vi "Periodic Tasks.vi"(8 "error in":errorcluster) -> ()   [LabVIEW 2013]
doc: "This VI runs in parallel to other tasks. It can contain as many user-defined periodic loops as you need. These can carry out PID or other sorts of timed response."
uses:
  <vilib>/Rock Robotics/SystemInterfaces/Utilities/FPGA_UtilitiesLED Source.ctl
  <vilib>/Rock Robotics/SystemInterfaces/Utilities/FPGA_UtilitiesLED State.ctl
  <vilib>/Rock Robotics/WPI/DriverStation/DriverStationLCD/WPI_DriverStationLCDLCDLine.ctl
  Robot Global Data.vi
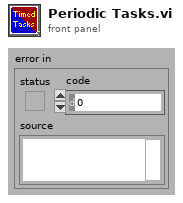
[diagram p1: front panel]
types:
  T1 = typedef "WPI_AnalogChannelDevRef.ctl" = cluster{"DevStatus":errorcluster, "Analog Module":T2, "Analog Channel":T3}
  T2 = typedef "FPGA_TypedefAnalogModule.ctl" = enum16{"Analog Module 1", "Analog Module 2"}
  T3 = typedef "FPGA_AIChannel.ctl" = enum8{"AI 1", "AI 2", "AI 3", "AI 4", "AI 5", "AI 6", "AI 7", "AI 8", "Invalid"}
  T4 = typedef "WPI_DigitalInputDevRef.ctl" = cluster{"DevStatus":errorcluster, "DIO Channel":T5, "Digital Module":T6}
  T5 = typedef "FPGA_DIOChannel.ctl" = enum8{"DIO 1", "DIO 2", "DIO 3", "DIO 4", "DIO 5", "DIO 6", "DIO 7", "DIO 8", "DIO 9", "DIO 10", "DIO 11", "DIO 12", "DIO 13", "DIO 14", "Invalid"}
  T6 = typedef "FPGA_TypedefDigitalModule.ctl" = enum16{"Digital Module 1", "Digital Module 2"}
  T7 = typedef "WPI_EncoderDevRef.ctl" = cluster{"DevStatus":errorcluster, "EncoderIndex":T8, "CounterIndex":T9, "DistancePerCount":dbl, "Decoding Type":T10}
  T8 = typedef "FPGA_EncoderIdx.ctl" = enum8{"Enc 0", "Enc 1", "Enc 2", "Enc 3", "Invalid"}
  T9 = typedef "FPGA_CounterCtrSystemIndex.ctl" = enum8{"Ctr 0", "Ctr 1", "Ctr 2", "Ctr 3", "Ctr 4", "Ctr 5", "Ctr 6", "Ctr 7", "Invalid"}
  T10 = typedef "WPI_EncoderType.ctl" = enum16{"1x", "2x", "4x"}
  T11 = cluster{"Winch Desired Location":dbl, "Winch Desired Location 2":dbl, "Winch Desired Location 3":dbl}
  T12 = typedef "FPGA_UtilitiesLED State.ctl" = enum16{"Off", "On", "Toggle"}
  T13 = typedef "FPGA_UtilitiesLED Source.ctl" = enum16{"User LED", "FPGA LED"}
  T14 = typedef "WPI_DriverStationLCDLCDLine.ctl" = enum16{"Main - Line 1", "User - Line 2", "User - Line 3", "User - Line 4", "User - Line 5", "User - Line 6"}
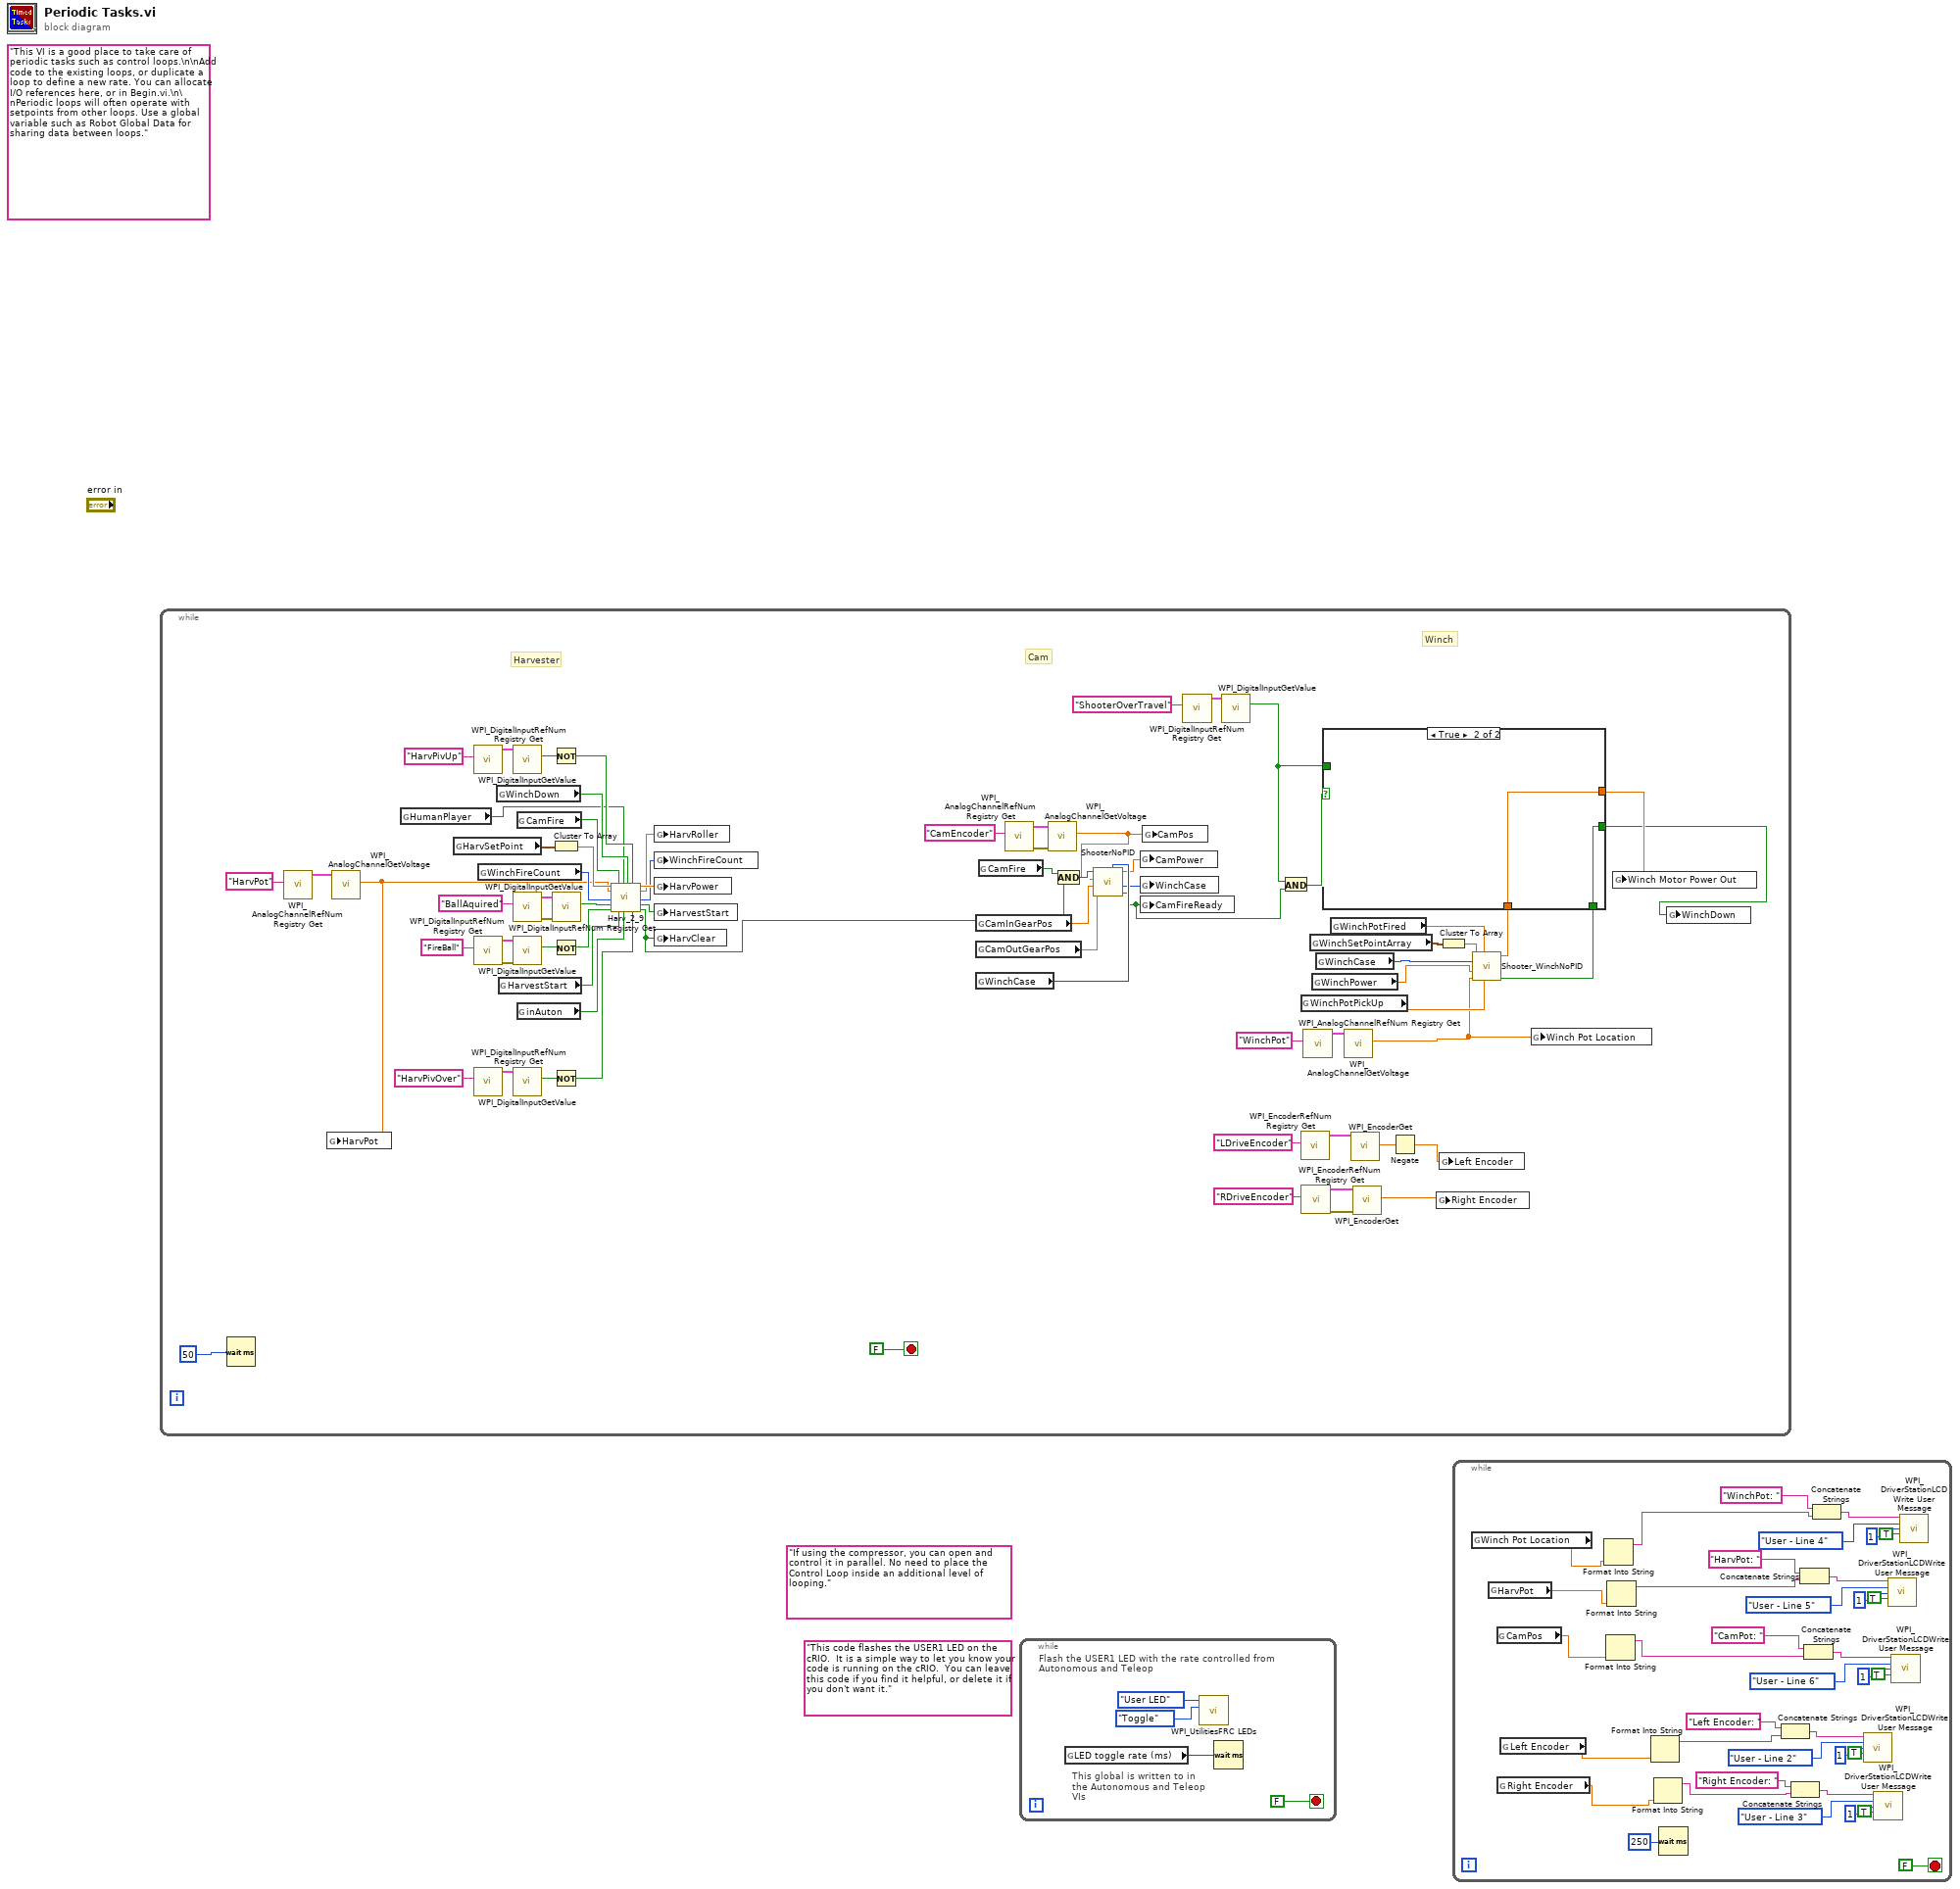
[diagram p0: block diagram]
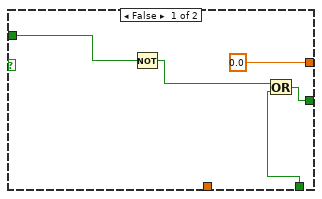
[diagram p2: hidden frame]
diagram:
  (unwired) "If using the compressor, you can open and control it in parallel. No need to place the Control Loop inside an additional level of looping."
  (unwired) "This code flashes the USER1 LED on the cRIO.  It is a simple way to let you know your code is running on the cRIO.  You can leave this code if you find it helpful, or delete it if you don't want it."
  (unwired) "This VI is a good place to take care of periodic tasks such as control loops.\n\nAdd code to the existing loops, or duplicate a loop to define a new rate. You can allocate I/O references here, or in Begin.vi.\n\nPeriodic loops will often operate with setpoints from other loops. Use a global variable such as Robot Global Data for sharing data between loops."
  n1 = while {
    stop <- FALSE stop-if-true
    # "Winch"
    # "Cam"
    # "Harvester"
    n2 = Wait (ms)(milliseconds to wait=u32 50) -> ()  [unwired: 1 out]
    n3 = call <vilib>:"WPI_AnalogChannelRefNum Registry Get.vi"("refnum name"="HarvPot") -> ("AIDeviceRef"=w71:T1)  [unwired: 9 in, 1 out]
    n4 = call <vilib>:"WPI_AnalogChannelGetVoltage.vi"("AIDeviceRef"=w71) -> ("Voltage"=w10:dbl)  [unwired: 8 in, 2 out]
    n5 = global write "Robot Global Data.vi" "HarvPot"(w10) -> ()
    n6 = global read "Robot Global Data.vi" "HumanPlayer"() -> (w1:bool)
    n7 = global read "Robot Global Data.vi" "HarvSetPoint"() -> (w38:cluster{"Out":dbl, "In":dbl, "Clear":dbl})
    n8 = call <vilib>:"WPI_DigitalInputRefNum Registry Get.vi"("refnum name"="HarvPivUp") -> ("DigitalInputDevRef"=w55:T4)  [unwired: 9 in, 1 out]
    n9 = call <vilib>:"WPI_DigitalInputRefNum Registry Get.vi"("refnum name"="FireBall") -> ("error out"=w44:errorcluster, "DigitalInputDevRef"=w45:T4)  [unwired: 9 in]
    n10 = call <vilib>:"WPI_DigitalInputRefNum Registry Get.vi"("refnum name"="HarvPivOver") -> ("DigitalInputDevRef"=w63:T4)  [unwired: 9 in, 1 out]
    n11 = global read "Robot Global Data.vi" "WinchFireCount"() -> (w13:i32)
    n12 = global read "Robot Global Data.vi" "WinchDown"() -> (w31:bool)
    n13 = global read "Robot Global Data.vi" "HarvestStart"() -> (w42:bool)
    n14 = call <vilib>:"WPI_DigitalInputGetValue.vi"("DigitalInputDevRef"=w55) -> ("Value"=w34:bool)  [unwired: 8 in, 2 out]
    n15 = call <vilib>:"WPI_DigitalInputRefNum Registry Get.vi"("refnum name"="BallAquired") -> ("error out"=w51:errorcluster, "DigitalInputDevRef"=w50:T4)  [unwired: 9 in]
    n16 = call <vilib>:"WPI_DigitalInputGetValue.vi"("error in (no error)"=w44, "DigitalInputDevRef"=w45) -> ("Value"=w41:bool)  [unwired: 7 in, 2 out]
    n17 = call <vilib>:"WPI_DigitalInputGetValue.vi"("DigitalInputDevRef"=w63) -> ("Value"=w36:bool)  [unwired: 8 in, 2 out]
    n18 = global read "Robot Global Data.vi" "CamFire"() -> (w43:bool)
    n19 = global read "Robot Global Data.vi" "inAuton"() -> (w15:bool)
    n20 = Not(x=w34) -> (.not. x?=w33:bool)
    n21 = Cluster To Array(cluster=w38) -> (array=w37:dbl[])
    n22 = call <vilib>:"WPI_DigitalInputGetValue.vi"("error in (no error)"=w51, "DigitalInputDevRef"=w50) -> ("Value"=w40:bool)  [unwired: 7 in, 2 out]
    n23 = Not(x=w41) -> (.not. x?=w39:bool)
    n24 = Not(x=w36) -> (.not. x?=w35:bool)
    n25 = call "Harv_2_9.vi"("HarvSetpoints"=w37, "HarvPot"=w10, "Count"=w13, "BallAcquired"=w40, "FireBallSen"=w39, "Fire"=w43, "Harvest"=w42, "HPButton"=w1, "inAuton?"=w15, "WinchDown"=w31, "HarvPivUP"=w33, "HarvPivPickupLim"=w35) -> ("HarvPower"=w48:dbl, "HarvRoller"=w47:dbl, "CountOut"=w12:i32, "HarvStart"=w32:bool, "HarvCleared"=w5:bool)  [unwired: 3 in]
    n26 = global write "Robot Global Data.vi" "HarvRoller"(w47) -> ()
    n27 = global write "Robot Global Data.vi" "WinchFireCount"(w12) -> ()
    n28 = global write "Robot Global Data.vi" "HarvPower"(w48) -> ()
    n29 = global write "Robot Global Data.vi" "HarvestStart"(w32) -> ()
    n30 = global write "Robot Global Data.vi" "HarvClear"(w5) -> ()
    n31 = global read "Robot Global Data.vi" "CamInGearPos"() -> (w20:dbl)
    n32 = global read "Robot Global Data.vi" "CamOutGearPos"() -> (w19:dbl)
    n33 = global read "Robot Global Data.vi" "WinchCase"() -> (w21:i32)
    n34 = global read "Robot Global Data.vi" "CamFire"() -> (w57:bool)
    n35 = call <vilib>:"WPI_AnalogChannelRefNum Registry Get.vi"("refnum name"="CamEncoder") -> ("error out"=w59:errorcluster, "AIDeviceRef"=w58:T1)  [unwired: 9 in]
    n36 = call <vilib>:"WPI_AnalogChannelGetVoltage.vi"("error in (no error)"=w59, "AIDeviceRef"=w58) -> ("Voltage"=w9:dbl)  [unwired: 7 in, 2 out]
    n37 = And(x=w57, y=w5) -> (x .and. y?=w22:bool)
    n38 = call "ShooterNoPID.vi"("WinchCaseIn"=w21, "InGearPosLow"=w19, "InGearPosHigh"=w20, "Pot"=w9, "Fire"=w22) -> ("There?"=w16:bool, "WinchCase"=w17:i32, "Power"=w18:dbl)  [unwired: 4 in]
    n39 = global write "Robot Global Data.vi" "CamPower"(w18) -> ()
    n40 = global write "Robot Global Data.vi" "WinchCase"(w17) -> ()
    n41 = global write "Robot Global Data.vi" "CamFireReady"(w16) -> ()
    n42 = global write "Robot Global Data.vi" "CamPos"(w9) -> ()
    n43 = call <vilib>:"WPI_DigitalInputRefNum Registry Get.vi"("refnum name"="ShooterOverTravel") -> ("DigitalInputDevRef"=w54:T4)  [unwired: 9 in, 1 out]
    n44 = call <vilib>:"WPI_DigitalInputGetValue.vi"("DigitalInputDevRef"=w54) -> ("Value"=w30:bool)  [unwired: 8 in, 2 out]
    n45 = And(x=w30, y=w16) -> (x .and. y?=w52:bool)
    n46 = global read "Robot Global Data.vi" "WinchPotPickUp"() -> (w14:dbl)
    n47 = call <vilib>:"WPI_EncoderRefNum Registry Get.vi"("refnum name"="LDriveEncoder") -> ("EncoderDevRef"=w65:T7)  [unwired: 9 in, 1 out]
    n48 = call <vilib>:"WPI_EncoderRefNum Registry Get.vi"("refnum name"="RDriveEncoder") -> ("error out"=w8:errorcluster, "EncoderDevRef"=w7:T7)  [unwired: 9 in]
    n49 = call <vilib>:"WPI_AnalogChannelRefNum Registry Get.vi"("refnum name"="WinchPot") -> ("AIDeviceRef"=w67:T1)  [unwired: 9 in, 1 out]
    n50 = global read "Robot Global Data.vi" "WinchSetPointArray"() -> (w27:T11)
    n51 = global read "Robot Global Data.vi" "WinchPower"() -> (w29:dbl)
    n52 = global read "Robot Global Data.vi" "WinchCase"() -> (w26:i32)
    n53 = global read "Robot Global Data.vi" "WinchPotFired"() -> (w2:dbl)
    n54 = call <vilib>:"WPI_AnalogChannelGetVoltage.vi"("AIDeviceRef"=w67) -> ("Voltage"=w11:dbl)  [unwired: 8 in, 2 out]
    n55 = call <vilib>:"WPI_EncoderGet.vi"("EncoderDevRef"=w65) -> ("Distance"=w4:dbl)  [unwired: 5 in, 5 out]
    n56 = call <vilib>:"WPI_EncoderGet.vi"("error in (no error)"=w8, "EncoderDevRef"=w7) -> ("Distance"=w6:dbl)  [unwired: 4 in, 5 out]
    n57 = Negate(x=w4) -> (-x=w3:dbl)
    n58 = global write "Robot Global Data.vi" "Right Encoder"(w6) -> ()
    n59 = Cluster To Array(cluster=w27) -> (array=w28:dbl[])
    n60 = global write "Robot Global Data.vi" "Left Encoder"(w3) -> ()
    n61 = call "Shooter_WinchNoPID.vi"("PickStartPos"=w14, "WinchFiredPos"=w2, "Winch Pot Location"=w11, "WinchPower"=w29, "selectedCase"=w26, "SetPointArray"=w28) -> ("isThere?"=w24:bool, "Winch Motor Power Out"=w23:dbl)  [unwired: 4 in]
    n62 = case shown="True" w52 {
      tunnel: [0.0 ("Winch Motor Power Out") w78] -> w61
      tunnel: [w76 w79] -> w25
      tunnel: w30 -> [w75 _]
      tunnel: w24 -> [w73 w79]
      tunnel: w23 -> [_ w78]
      frame False {
        n63 = Not(x=w75) -> (.not. x?=w74:bool)
        n64 = Or(x=w74, y=w73) -> (x .or. y?=w76:bool)
      }
      frame True {
      }
    }
    n65 = global write "Robot Global Data.vi" "Winch Pot Location"(w11) -> ()
    n66 = global write "Robot Global Data.vi" "Winch Motor Power Out"(w61) -> ()
    n67 = global write "Robot Global Data.vi" "WinchDown"(w25) -> ()
  }
  n68 = while {
    stop <- FALSE stop-if-true
    # "This global is written to in the Autonomous and Teleop VIs"
    # "Flash the USER1 LED with the rate controlled from Autonomous and Teleop"
    n69 = global read "Robot Global Data.vi" "LED toggle rate (ms)"() -> (w80:u32)
    n70 = call <vilib>:"WPI_UtilitiesFRC LEDs.vi"("State"=FPGA_UtilitiesLED_State."Toggle", "LED Type"=FPGA_UtilitiesLED_Source."User LED") -> ()  [unwired: 1 in, 9 out]
    n71 = Wait (ms)(milliseconds to wait=w80) -> ()  [unwired: 1 out]
  }
  n72 = while {
    stop <- FALSE stop-if-true
    n73 = global read "Robot Global Data.vi" "Winch Pot Location"() -> (w89:dbl)
    n74 = global read "Robot Global Data.vi" "HarvPot"() -> (w88:dbl)
    n75 = global read "Robot Global Data.vi" "CamPos"() -> (w90:dbl)
    n76 = global read "Robot Global Data.vi" "Right Encoder"() -> (w86:dbl)
    n77 = global read "Robot Global Data.vi" "Left Encoder"() -> (w87:dbl)
    n78 = Format Into String(w89) -> (resulting string=w106:string)  [unwired: 3 in, 1 out]
    n79 = Format Into String(w90) -> (resulting string=w91:string)  [unwired: 3 in, 1 out]
    n80 = Format Into String(w88) -> (resulting string=w100:string)  [unwired: 3 in, 1 out]
    n81 = Format Into String(w87) -> (resulting string=w98:string)  [unwired: 3 in, 1 out]
    n82 = Format Into String(w86) -> (resulting string=w97:string)  [unwired: 3 in, 1 out]
    n83 = Wait (ms)(milliseconds to wait=u32 250) -> ()  [unwired: 1 out]
    n84 = Concatenate Strings("Left Encoder: ", w98) -> (w116:string)
    n85 = Concatenate Strings("Right Encoder: ", w97) -> (w115:string)
    n86 = Concatenate Strings("HarvPot: ", w100) -> (w101:string)
    n87 = Concatenate Strings("CamPot: ", w91) -> (w96:string)
    n88 = Concatenate Strings("WinchPot: ", w106) -> (w111:string)
    n89 = call <vilib>:"WPI_DriverStationLCDWrite User Message.vi"("line text"=w116, "line"=WPI_DriverStationLCDLCDLine."User - Line 2", "starting column"=i8 1, "clear line before write (T)"=TRUE) -> ()  [unwired: 1 in, 11 out]
    n90 = call <vilib>:"WPI_DriverStationLCDWrite User Message.vi"("line text"=w115, "line"=WPI_DriverStationLCDLCDLine."User - Line 3", "starting column"=i8 1, "clear line before write (T)"=TRUE) -> ()  [unwired: 1 in, 11 out]
    n91 = call <vilib>:"WPI_DriverStationLCDWrite User Message.vi"("line text"=w101, "line"=WPI_DriverStationLCDLCDLine."User - Line 5", "starting column"=i8 1, "clear line before write (T)"=TRUE) -> ()  [unwired: 1 in, 11 out]
    n92 = call <vilib>:"WPI_DriverStationLCDWrite User Message.vi"("line text"=w96, "line"=WPI_DriverStationLCDLCDLine."User - Line 6", "starting column"=i8 1, "clear line before write (T)"=TRUE) -> ()  [unwired: 1 in, 11 out]
    n93 = call <vilib>:"WPI_DriverStationLCDWrite User Message.vi"("line text"=w111, "line"=WPI_DriverStationLCDLCDLine."User - Line 4", "starting column"=i8 1, "clear line before write (T)"=TRUE) -> ()  [unwired: 1 in, 11 out]
  }
